vi "Keysight BenchVue Data Viewer.vi"() -> ()   [LabVIEW 2015]
uses:
  <vilib>/addons/_office/excel.llb/Excel Get Data ([str]).vi
  <vilib>/Utility/NIReport.llb/NI_report.lvclass
  <vilib>/Utility/NIReport.llb/Excel/NI_Excel.lvclass
  <vilib>/addons/_office/NI_ReportGenerationToolkit.lvlib
panel:
  in  "정지 버튼":bool
  out "Delta x":dbl
  out "XY 그래프":cluster{dbl[], dbl[]}[](graph)
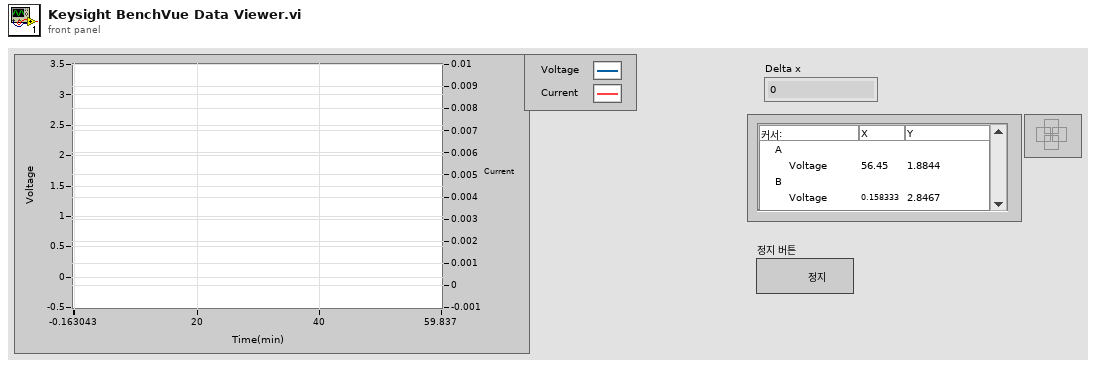
[diagram p1: front panel]
types:
  T1 = enum16{"maximized", "minimized", "normal", "no change"}
  T2 = enum16{"Standard Report", "HTML", "Word", "Excel"}
  T3 = typedef "LVCursorListTypeDef.ctl" = cluster{"Name":string, "Color":u32, "Style":u8, "Point Style":u8, "Name Visible":bool, "Allow Drag":bool, "Cursor Mode":u32, "Plot":i32, "Index":i32, "Position":cluster{"X":dbl, "Y":dbl}, "X Scale":u32, "Y Scale":u32, "Watch Plots":i32[], "Watch All Plots":bool, "Plot Area":i32, "Label Offset":cluster{"X":dbl, "Y":dbl}}[]
  T4 = cluster{"Name":string, "Color":u32, "Style":u8, "Point Style":u8, "Name Visible":bool, "Allow Drag":bool, "Cursor Mode":u32, "Plot":i32, "Index":i32, "Position":cluster{"X":dbl, "Y":dbl}, "X Scale":u32, "Y Scale":u32, "Watch Plots":i32[], "Watch All Plots":bool, "Plot Area":i32, "Label Offset":cluster{"X":dbl, "Y":dbl}}
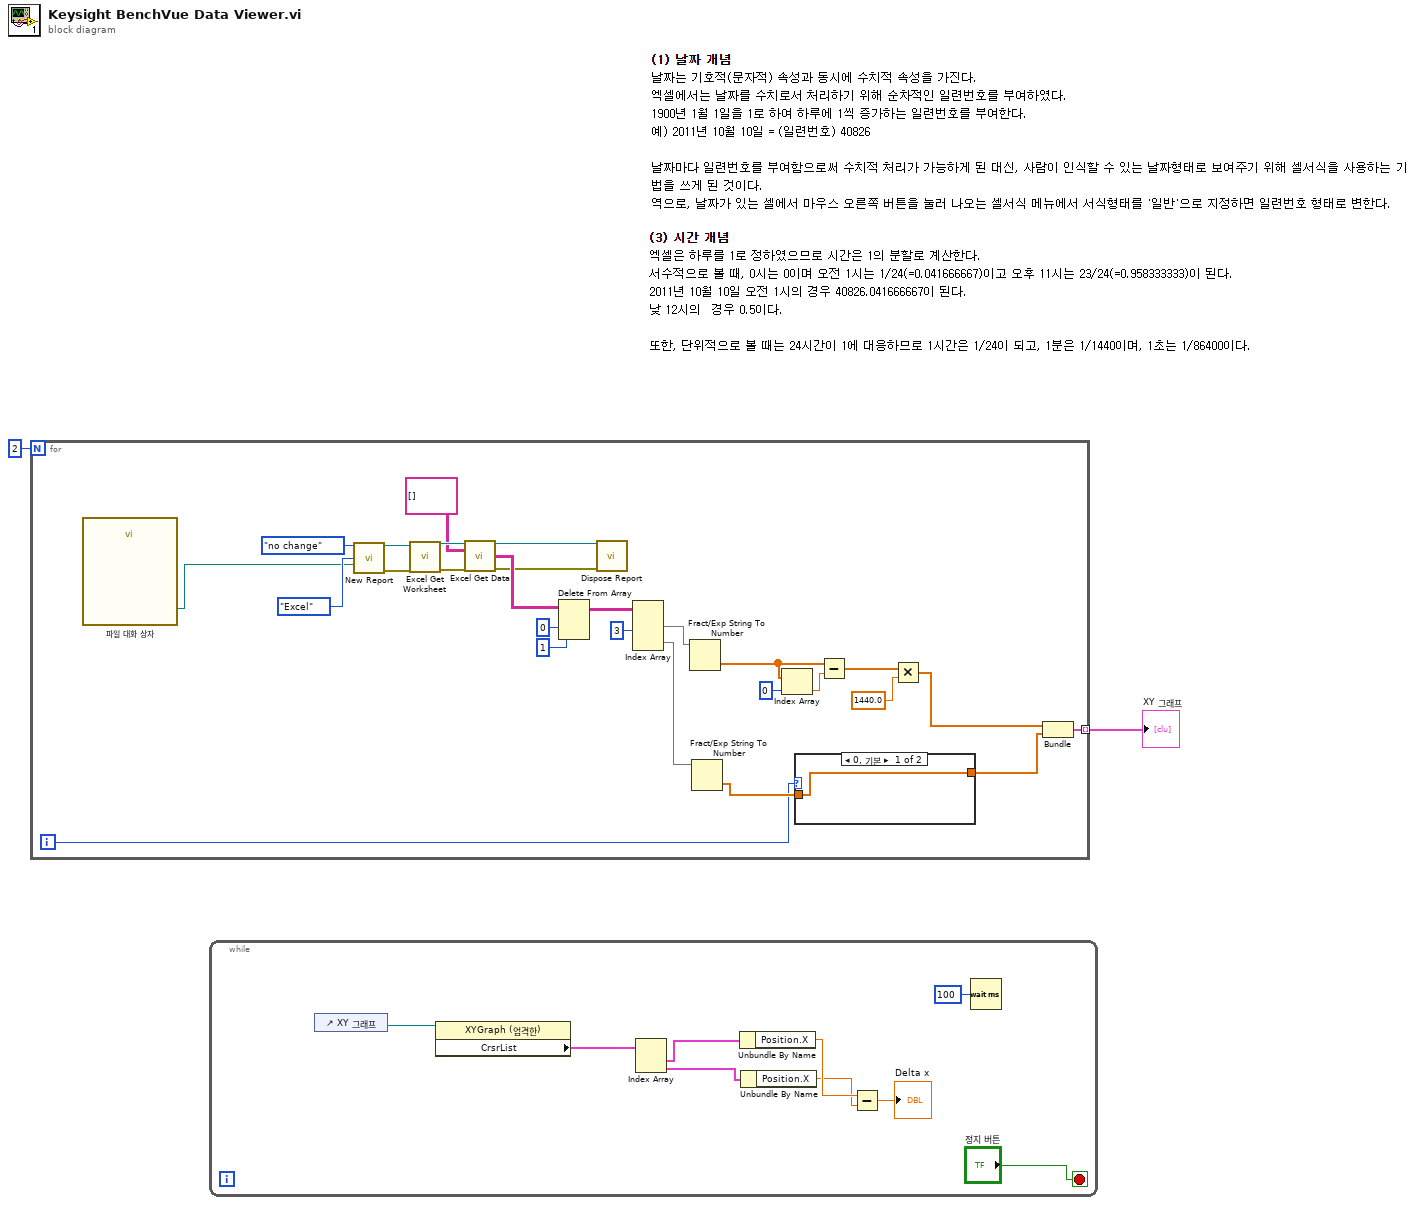
[diagram p0: block diagram]
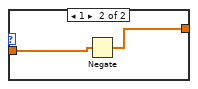
[diagram p2: hidden frame]
diagram:
  n1 = for {
    N: 2 -> [_]
    tunnel: [w4] -> w1 mode=indexing
    i -> [w3]
    n2 = call "파일 대화 상자"() -> ("selected path"=w24:path)  [unwired: 12 in, 3 out]
    n3 = call <vilib>:"New Report.vi"("window state (normal)"=T1."no change", "report type"=T2."Excel", "template (empty)"=w24) -> ("report out"=w29:refnum<class "NI_report.lvclass">, "error out"=w28:errorcluster)  [unwired: 11 in]
    n4 = call <vilib>:"Excel Get Worksheet.vi"("report in"=w29, "error in (no error)"=w28) -> ("report out"=w27:refnum<class "NI_report.lvclass">, "error out"=w26:errorcluster)  [unwired: 12 in]
    n5 = call-poly <vilib>:"Excel Get Data.vi"("report in"=w27, "data type"=string[][] [], "error in (no error)"=w26) -> ("report out"=w8:refnum<class "NI_report.lvclass">, "data"=w21:string[][], "error out"=w7:errorcluster)  [unwired: 10 in]
    n6 = Delete From Array(array=w21, length=1 ("길이"), index (row)=0 ("인덱스 (행)")) -> (array with subset deleted=w18:string[][])  [unwired: 1 in, 1 out]
    n7 = call-dynamic "Dispose Report.vi"("report in"=w8, "error in (no error)"=w7) -> ()  [unwired: 13 in, 1 out]
    n8 = Index Array(array=w18, index (col) #1=3 ("비활성화된 인덱스 (열)")) -> (element #1=w16:string[], element #2=w10:string[])  [unwired: 3 in]
    n9 = Fract/Exp String To Number(string=w16) -> (number=w13:dbl[])  [unwired: 3 in, 1 out]
    n10 = Fract/Exp String To Number(string=w10) -> (number=w6:dbl[])  [unwired: 3 in, 1 out]
    n11 = Index Array(array=w13, index=0 ("인덱스")) -> (element=w15:dbl)
    n12 = case shown="0, 기본" w3 {
      tunnel: w6 -> [w30 w32]
      tunnel: [w30 w31] -> w5
      frame 0, Default {
      }
      frame 1 {
        n13 = Negate(x=w32) -> (-x=w31:dbl[])
      }
    }
    n14 = Subtract(x=w13, y=w15) -> (x-y=w12:dbl[])
    n15 = Multiply(x=w12, y=1440.0) -> (x*y=w9:dbl[])
    n16 = Bundle(w9, w5) -> (w4:cluster{dbl[], dbl[]})  [unwired: 1 in]
  }
  "XY 그래프" <- w1
  n17 = while {
    stop <- "정지 버튼" stop-if-true
    n18 = control-ref of="XY 그래프"() -> (w41:refnum<vi>)
    n19 = property class="XYGraph (엄격한)"(reference=w41) -> ("CrsrList"=w37:T3)  [unwired: 1 in, 2 out]
    n20 = Index Array(array=w37) -> (element #1=w36:T4, element #2=w35:T4)  [unwired: 2 in]
    n21 = Unbundle By Name(w36) -> ("Position.X"=w34:dbl)
    n22 = Unbundle By Name(w35) -> ("Position.X"=w33:dbl)
    n23 = Subtract(x=w34, y=w33) -> (x-y=→"Delta x":dbl)
    n24 = Wait (ms)(milliseconds to wait=u32 100 ("대기 시간(ms)")) -> ()  [unwired: 1 out]
  }
